vi "CreateNewParamTestCase.vi"(8 "error in (no error)":errorcluster, 10 "Path":path, 11 "Application":refnum<vi>) -> (0 "error out":errorcluster)   [LabVIEW 2020]
uses:
  <vilib>/Utility/error.llb/Error Cluster From Error Code.vi
  <vilib>/ErrorRing/Error Ring.xnode
  <resource>/Framework/Providers/LUnit Project Provider.lvlib
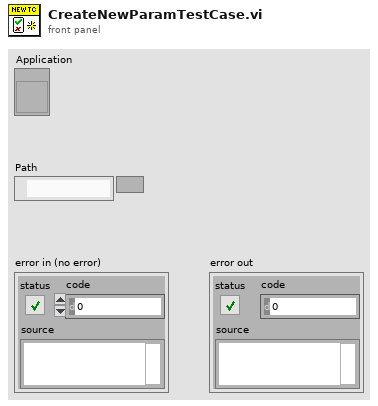
[diagram p1: front panel]
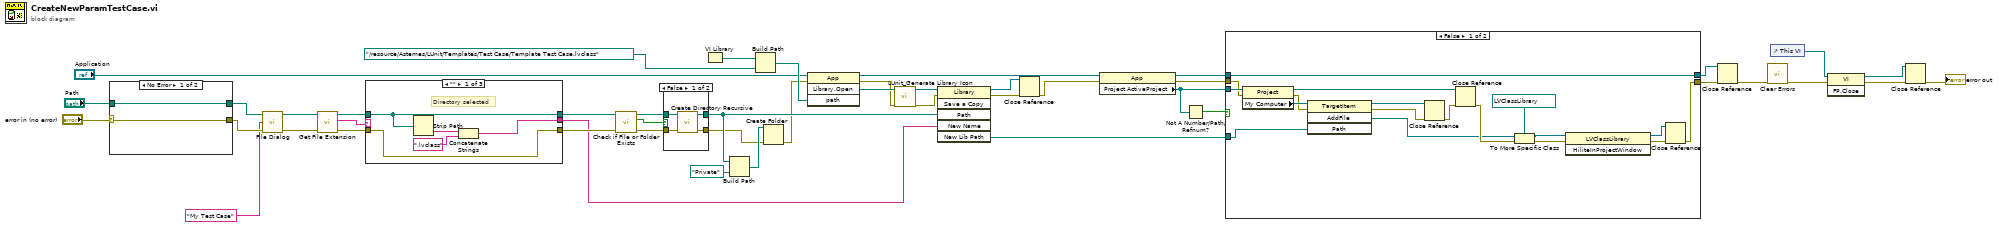
[diagram p0: block diagram]
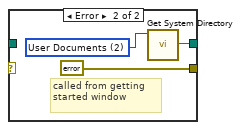
[diagram p2: hidden frame]
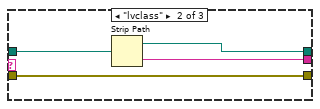
[diagram p3: hidden frame]
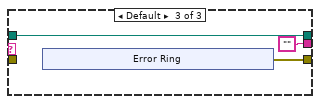
[diagram p4: hidden frame]
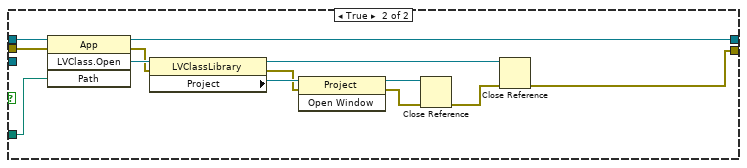
[diagram p6: hidden frame]
diagram:
  n1 = case shown="No Error" "error in (no error)" {
    selector: "error in (no error)" -> [w48 _]
    tunnel: [w48 errorcluster {"status"=FALSE, "code"=0, "source"=""} ("error IO")] -> w17
    tunnel: [w47 w49] -> w18
    tunnel: "Path" -> [w47 _]
    frame No Error {
    }
    frame Error {
      w50 = 2 items=["User Home"=0, "User Desktop"=1, "User Documents"=2, "User Application Data"=3, "User Preferences"=4, "User Temporary"=5, "Public Documents"=6, "Public Application Data"=7, "Public Preferences"=8, "Public Cache"=13, "System Core Libraries"=9, "System Installed Libraries"=10, "Application Files"=11, "Boot Volume Root"=12] ("system directory type")
      # "called from getting started window"
      n2 = call <vilib>:"Get System Directory.vi"("system directory type"=w50) -> ("system directory"=w49:path)  [unwired: 10 in]
    }
  }
  n3 = call "File Dialog"("start path"=w18, "default name"="My Test Case", "error in"=w17) -> ("selected path"=w43:path, "error out"=w16:errorcluster)  [unwired: 9 in, 2 out]
  n4 = call <vilib>:"Get File Extension.vi"("error in (no error)"=w16, "file"=w43) -> ("error out"=w46:errorcluster, "lowercase file extension"=w45:string, "dup file"=w44:path)  [unwired: 5 in, 2 out]
  n5 = case shown="\"\"" w45 {
    tunnel: w46 -> [w52 w57 _]
    tunnel: w44 -> [w53 w60 w61]
    tunnel: [w52 w57 w63] -> w41
    tunnel: [w54 w59 "" ("name")] -> w37
    tunnel: [w53 w58 w61] -> w42
    frame "" {
      # "Directory selected"
      n6 = Strip Path(path=w53) -> (name=w56:string)  [unwired: 1 out]
      n7 = Concatenate Strings(w56, ".lvclass" ("string")) -> (w54:string)
    }
    frame "lvclass" {
      n8 = Strip Path(path=w60) -> (stripped path=w58:path, name=w59:string)
    }
    frame Default {
      n9 = xnode "Error Ring"() -> ("error out"=w63:errorcluster)
    }
  }
  n10 = call <vilib>:"Check if File or Folder Exists.vi"("error in (no error)"=w41, "path"=w42) -> ("error out"=w40:errorcluster, "file or folder exists?"=w38:bool, "dup path"=w39:path)  [unwired: 7 in]
  n11 = case shown="False" w38 {
    tunnel: w40 -> [w71 w72]
    tunnel: w39 -> [w70 w73]
    tunnel: [w69 w73] -> w10
    tunnel: [w68 w72] -> w9
    frame False {
      n12 = call <vilib>:"Create Directory Recursive.vi"("error in (no error)"=w71, "directory"=w70) -> ("error out"=w68:errorcluster, "directory copy"=w69:path)  [unwired: 3 in, 1 out]
    }
    frame True {
    }
  }
  n13 = VI Library() -> (path=w30:path)
  n14 = Build Path(base path=w10, name or relative path=path "Private") -> (appended path=w12:path)
  n15 = Build Path(base path=w30, name or relative path=path "../resource/Astemes/LUnit/Templates/Test Case/Template Test Case.lvclass") -> (appended path=w28:path)
  n16 = Create Folder(path (use dialog)=w12, error in=w9) -> (error out=w8:errorcluster)  [unwired: 1 in, 2 out]
  n17 = invoke class="App" method="Library.Open"(reference="Application", error in=w8, "path"=w28) -> (reference out=w5:refnum<vi>, error out=w1:errorcluster, "Open Library"=w4:refnum<vi>)  [unwired: 1 in, 1 out]
  n18 = call <resource>:"LUnit_Generate Library Icon.vi"("error in (no error)"=w1, "Library Refnum in"=w4) -> ("error out"=w2:errorcluster, "Library Refnum out"=w3:refnum<vi>)  [unwired: 8 in]
  n19 = invoke class="Library" method="Save a Copy"(reference=w3, error in=w2, "Path"=w10, "New Name"=w37) -> (reference out=w26:refnum<vi>, error out=w25:errorcluster, "New Lib Path"=w7:path)  [unwired: 2 in, 3 out]
  n20 = Close Reference(reference=w26, error in (no error)=w25) -> (error out=w6:errorcluster)
  n21 = property class="App"(reference=w5, error in=w6) -> (reference out=w33:refnum<vi>, error out=w34:errorcluster, "Project.ActiveProject"=w35:refnum<vi>)
  n22 = Not A Number/Path/Refnum?(number/path/refnum=w35) -> (NaN/Path/Refnum?=w36:bool)
  n23 = case shown="False" w36 {
    tunnel: w35 -> [w91 _]
    tunnel: w34 -> [w89 w95]
    tunnel: w7 -> [w83 w93]
    tunnel: [w78 w92] -> w31
    tunnel: w33 -> [w82 w96]
    tunnel: [w82 w94] -> w32
    frame False {
      n24 = property class="Project"(reference=w91, error in=w89) -> (reference out=w85:refnum<vi>, error out=w88:errorcluster, "My Computer"=w90:refnum<vi>)
      n25 = invoke class="TargetItem" method="AddFile"(reference=w90, error in=w88, "Path"=w83) -> (reference out=w86:refnum<vi>, error out=w87:errorcluster, "AddFile"=w74:refnum<vi>)  [unwired: 1 in, 1 out]
      n26 = Close Reference(reference=w86, error in (no error)=w87) -> (error out=w84:errorcluster)
      n27 = Close Reference(reference=w85, error in (no error)=w84) -> (error out=w81:errorcluster)
      n28 = To More Specific Class(target class=refnum<vi> refnum ("reference"), reference=w74, error in=w81) -> (specific class reference=w75:refnum<vi>, error out=w77:errorcluster)
      n29 = invoke class="LVClassLibrary" method="HiliteInProjectWindow"(reference=w75, error in=w77) -> (reference out=w79:refnum<vi>, error out=w80:errorcluster)  [unwired: 1 in, 1 out]
      n30 = Close Reference(reference=w79, error in (no error)=w80) -> (error out=w78:errorcluster)
    }
    frame True {
      n31 = invoke class="App" method="LVClass.Open"(reference=w96, error in=w95, "Path"=w93) -> (reference out=w94:refnum<vi>, error out=w103:errorcluster, "LVClass.Open"=w104:refnum<vi>)  [unwired: 1 in, 1 out]
      n32 = property class="LVClassLibrary"(reference=w104, error in=w103) -> (reference out=w102:refnum<vi>, error out=w100:errorcluster, "Project"=w101:refnum<vi>)
      n33 = invoke class="Project" method="Open Window"(reference=w101, error in=w100) -> (reference out=w99:refnum<vi>, error out=w98:errorcluster)  [unwired: 1 in, 1 out]
      n34 = Close Reference(reference=w99, error in (no error)=w98) -> (error out=w97:errorcluster)
      n35 = Close Reference(reference=w102, error in (no error)=w97) -> (error out=w92:errorcluster)
    }
  }
  n36 = Close Reference(reference=w32, error in (no error)=w31) -> (error out=w27:errorcluster)
  n37 = call <vilib>:"Clear Errors.vi"("error in (no error)"=w27) -> ("error out"=w20:errorcluster)  [unwired: 5 in, 1 out]
  n38 = control-ref of="This VI"() -> (w24:refnum<vi>)
  n39 = invoke class="VI" method="FP.Close"(reference=w24, error in=w20) -> (reference out=w22:refnum<vi>, error out=w21:errorcluster)  [unwired: 1 in, 1 out]
  n40 = Close Reference(reference=w22, error in (no error)=w21) -> (error out=→"error out":errorcluster)
